vi "lidarPos.vi"(7 "robotPos":cluster{"xPos":dbl, "yPos":dbl, "theta":dbl}, 8 "angle deviation":dbl, 9 "landmarks":cluster{dbl, dbl}[](array[cluster]), 10 "corners":cluster{dbl, dbl}[](array[cluster]), 11 "acceptance threshold":dbl) -> (2 "lidarPos":cluster{"xPos":dbl, "yPos":dbl, "theta":dbl})   [LabVIEW 2016]
panel:
  out "associated landmarks":cluster{cluster{dbl, dbl}, cluster{dbl, dbl}}
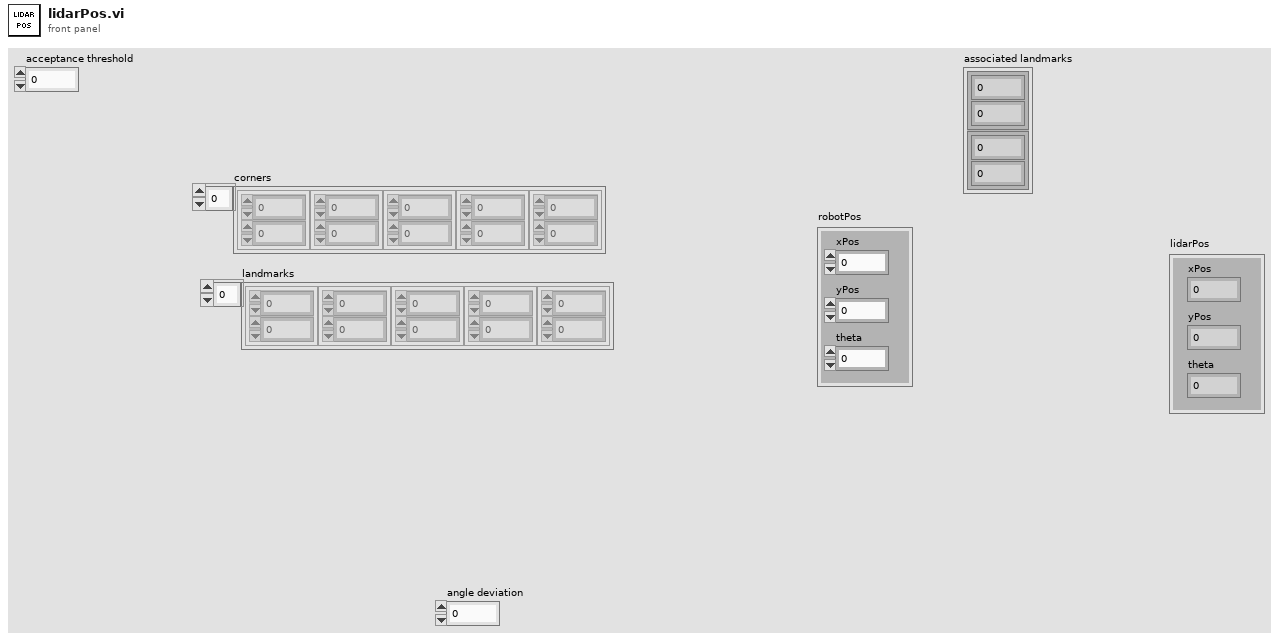
[diagram p1: front panel]
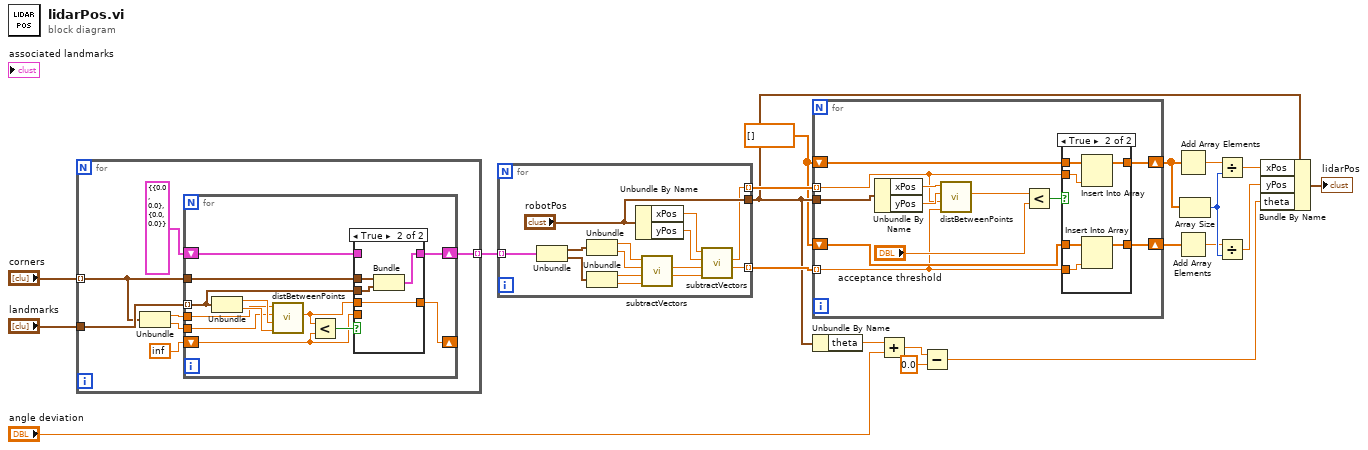
[diagram p0: block diagram]
diagram:
  w6 = dbl[] []
  n1 = for {
    tunnel: "corners" -> [w23] mode=indexing
    tunnel: "landmarks" -> [w27]
    tunnel: [w21] -> w18 mode=indexing
    n2 = Unbundle(w23) -> (w25:dbl, w26:dbl)
    n3 = for {
      tunnel: w27 -> [w35] mode=indexing
      tunnel: w26 -> [w30]
      tunnel: w25 -> [w29]
      shift-right: [w38] -> _
      shift-left: inf -> [w37]
      tunnel: w23 -> [w36]
      shift-right: [w34] -> w21
      shift-left: cluster{cluster{dbl, dbl}, cluster{dbl, dbl}} {{0.0, 0.0}, {0.0, 0.0}} -> [w33]
      n4 = Unbundle(w35) -> (w31:dbl, w32:dbl)
      n5 = call "distBetweenPoints.vi"("y2"=w32, "x2"=w31, "y1"=w30, "x1"=w29) -> ("d"=w28:dbl)  [unwired: 7 in]
      n6 = Less?(x=w28, y=w37) -> (x < y?=w39:bool)
      n7 = case shown="True" w39 {
        tunnel: [w41 w42] -> w38
        tunnel: w37 -> [w41 _]
        tunnel: w36 -> [_ w45]
        tunnel: w35 -> [_ w44]
        tunnel: [w40 w43] -> w34
        tunnel: w33 -> [w40 _]
        tunnel: w28 -> [_ w42]
        frame False {
        }
        frame True {
          n8 = Bundle(w45, w44) -> (w43:cluster{cluster{dbl, dbl}, cluster{dbl, dbl}})  [unwired: 1 in]
        }
      }
    }
  }
  n9 = for {
    tunnel: w18 -> [w59] mode=indexing
    tunnel: ["robotPos"] -> w12
    tunnel: [w51] -> w14 mode=indexing
    tunnel: [w50] -> w13 mode=indexing
    n10 = Unbundle(w59) -> (w58:cluster{dbl, dbl}, w57:cluster{dbl, dbl})
    n11 = Unbundle(w58) -> (w53:dbl, w52:dbl)
    n12 = Unbundle(w57) -> (w55:dbl, w54:dbl)
    n13 = Unbundle By Name("robotPos") -> ("xPos"=w49:dbl, "yPos"=w48:dbl)
    n14 = call "subtractVectors.vi"("y2"=w54, "x2"=w55, "y1"=w52, "x1"=w53) -> ("y"=w46:dbl, "x"=w47:dbl)  [unwired: 6 in]
    n15 = call "subtractVectors.vi"("y2"=w46, "x2"=w47, "y1"=w48, "x1"=w49) -> ("y"=w50:dbl, "x"=w51:dbl)  [unwired: 6 in]
  }
  n16 = for {
    tunnel: w14 -> [w64] mode=indexing
    tunnel: w13 -> [w60] mode=indexing
    tunnel: w12 -> [w71]
    shift-right: [w63] -> w4
    shift-left: w6 -> [w65]
    shift-right: [w61] -> w5
    shift-left: w6 -> [w62]
    n17 = Unbundle By Name(w71) -> ("xPos"=w70:dbl, "yPos"=w69:dbl)
    n18 = call "distBetweenPoints.vi"("y2"=w60, "x2"=w64, "y1"=w69, "x1"=w70) -> ("d"=w68:dbl)  [unwired: 7 in]
    n19 = Less?(x=w68, y="acceptance threshold") -> (x < y?=w66:bool)
    n20 = case shown="True" w66 {
      tunnel: [w73 w79] -> w63
      tunnel: w65 -> [w73 w78]
      tunnel: w64 -> [_ w77]
      tunnel: w62 -> [w72 w76]
      tunnel: [w72 w75] -> w61
      tunnel: w60 -> [_ w74]
      frame False {
      }
      frame True {
        n21 = Insert Into Array(array=w78, new element=w77) -> (w79:dbl[])  [unwired: 1 in]
        n22 = Insert Into Array(array=w76, new element=w74) -> (w75:dbl[])  [unwired: 1 in]
      }
    }
  }
  n23 = Unbundle By Name(w12) -> ("theta"=w16:dbl)
  n24 = Add(x=w16, y="angle deviation") -> (x+y=w3:dbl)
  n25 = Subtract(x=w3, y=0.0) -> (x-y=w1:dbl)
  n26 = Add Array Elements(numeric array=w4) -> (sum=w11:dbl)
  n27 = Add Array Elements(numeric array=w5) -> (sum=w9:dbl)
  n28 = Array Size(array=w4) -> (size(s)=w10:i32)
  n29 = Divide(x=w11, y=w10) -> (x/y=w8:dbl)
  n30 = Divide(x=w9, y=w10) -> (x/y=w7:dbl)
  n31 = Bundle By Name(cluster=w12, "xPos"=w8, "yPos"=w7, "theta"=w1) -> (→"lidarPos":cluster{"xPos":dbl, "yPos":dbl, "theta":dbl})
